vi "LVJSON Flatten.vi"(8 "error in (no error)":errorcluster, 9 "Enums as string? (F)":bool, 10 "Root Path ([]=Root)":string[](array[string]), 11 "Variant in":variant) -> (0 "error out":errorcluster, 3 "Root Element out":T1)   [LabVIEW 2018, in "labview_json.lvlib"]
uses:
  labview_json.lvlib
  <vilib>/Utility/Data Type/NI_Data Type.lvlib
  Element Type.ctl
  <vilib>/Utility/error.llb/Error Cluster From Error Code.vi
  <vilib>/ErrorRing/Error Ring.xnode
  Element.ctl
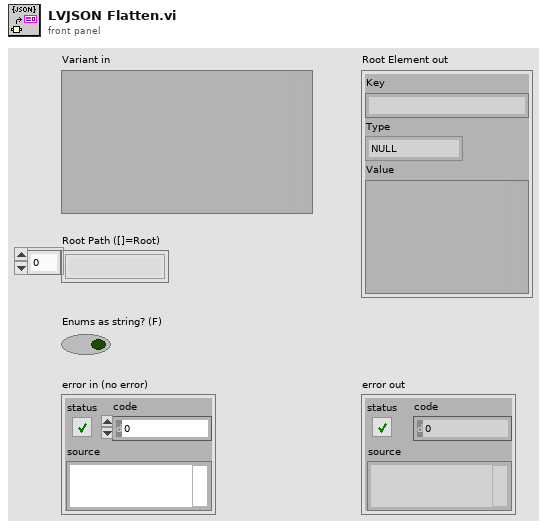
[diagram p1: front panel]
types:
  T1 = typedef "labview_json.lvlib/Element.ctl" = cluster{"Key":string, "Type":T2, "Value":variant}
  T2 = typedef "labview_json.lvlib/Element Type.ctl" = enum8{"NULL", "BOOL", "INT", "UINT", "FLOAT", "STRING", "ARRAY", "OBJECT", "SKIP"}
  T3 = typedef "NI_Data Type.lvlib/Data Type.ctl" = enum8{"Invalid Type", "Void", "I8", "I16", "I32", "I64", "U8", "U16", "U32", "U64", "Single Float", "Double Float", "Extended Float", "Single Complex", "Double Complex", "Extended Complex", "Enum U8", "Enum U16", "Enum U32", "Enum U64", "Single Float With Unit", "Double Float With Unit", "Extended Float With Unit", "Single Complex with Unit", "Double Complex with Unit", "Extended Complex with Unit", "Boolean", "String", "Path", "Picture", "Tag", "Array", "Cluster", "Variant", "LV Variant", "Waveform", "Timestamp", "Digital Waveform", "Digital Data", "ExpressData", "Refnum", "External Data", "VI", "Poly VI", "LabVIEW Class Instance", "Fixed Point", "Set Collection", "Map Collection"}
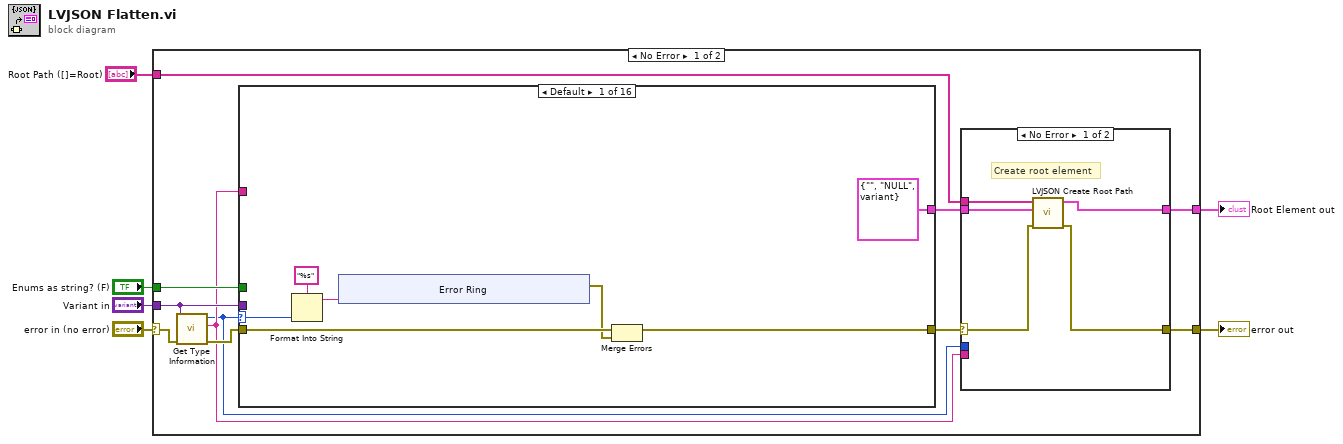
[diagram p0: block diagram]
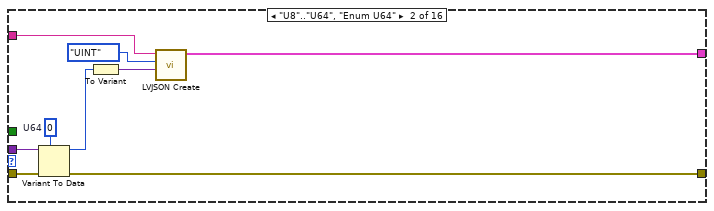
[diagram p2: hidden frame]
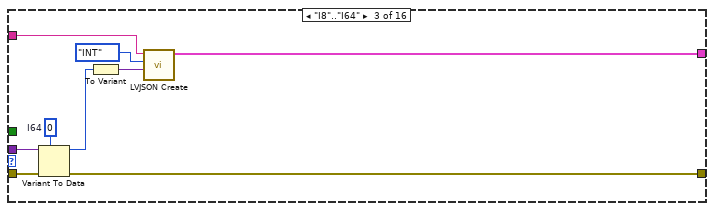
[diagram p3: hidden frame]
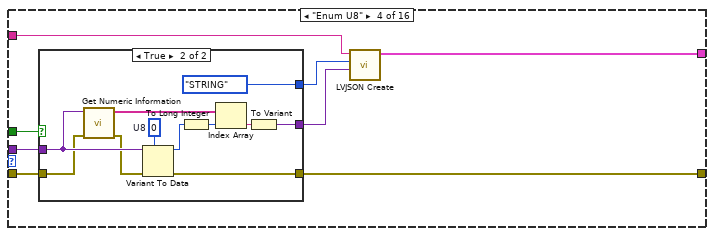
[diagram p4: hidden frame]
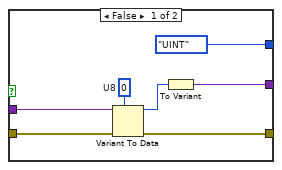
[diagram p5: hidden frame]
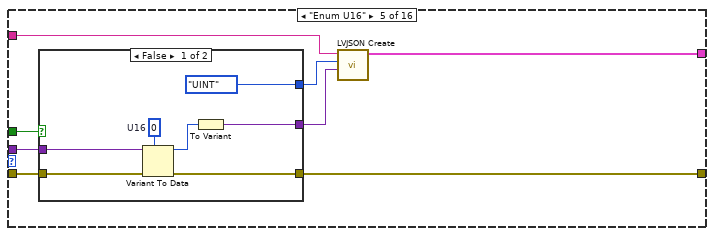
[diagram p6: hidden frame]
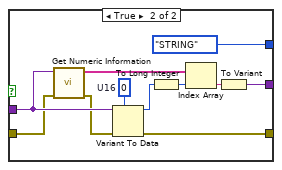
[diagram p7: hidden frame]
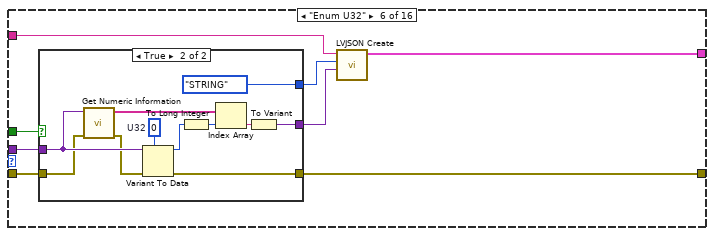
[diagram p8: hidden frame]
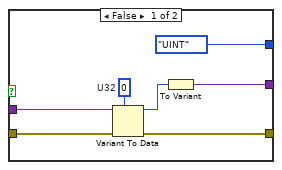
[diagram p9: hidden frame]
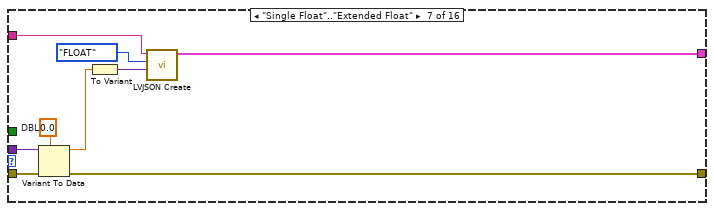
[diagram p10: hidden frame]
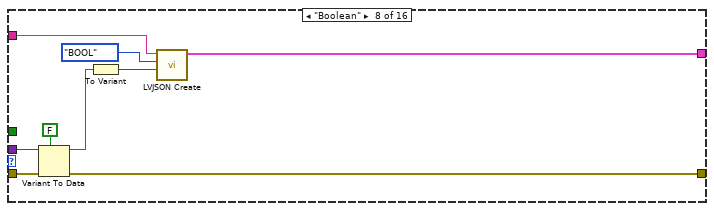
[diagram p11: hidden frame]
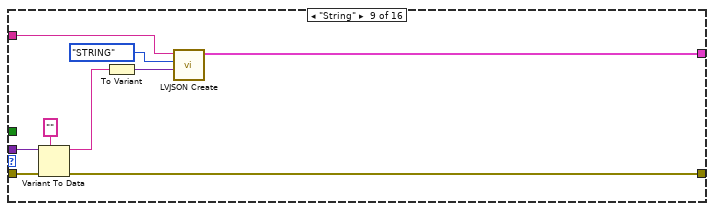
[diagram p12: hidden frame]
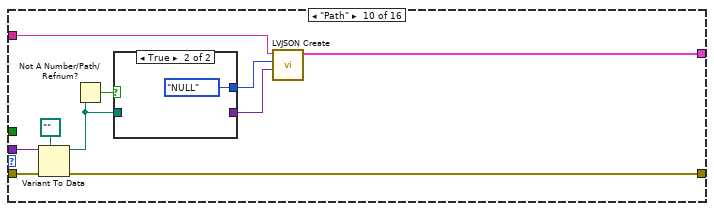
[diagram p13: hidden frame]
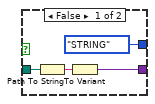
[diagram p14: hidden frame]
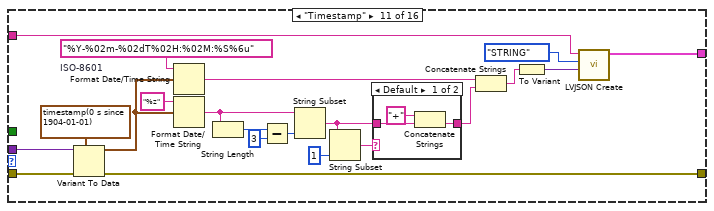
[diagram p15: hidden frame]
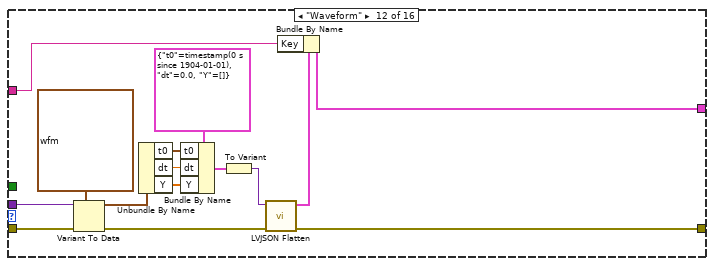
[diagram p17: hidden frame]
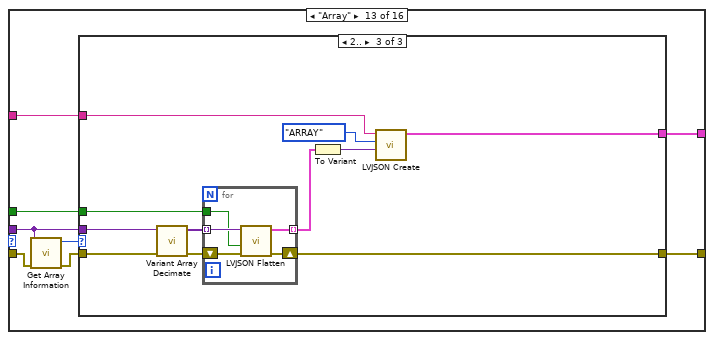
[diagram p18: hidden frame]
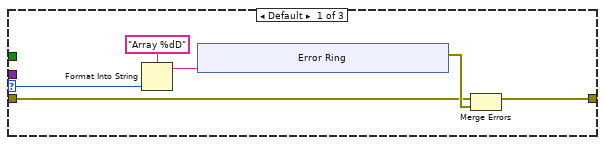
[diagram p19: hidden frame]
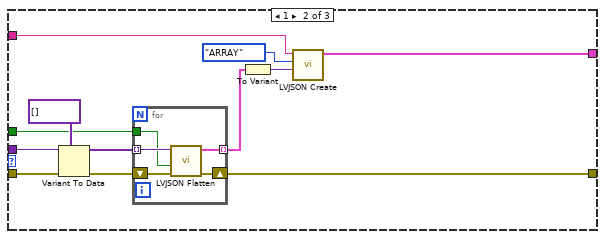
[diagram p20: hidden frame]
diagram:
  n1 = case shown="No Error" "error in (no error)" {
    selector: "error in (no error)" -> [w17 w322]
    tunnel: "Variant in" -> [w15 _]
    tunnel: [w12 w322] -> w4
    tunnel: [w10 _] -> w2
    tunnel: "Enums as string? (F)" -> [w14 _]
    tunnel: "Root Path ([]=Root)" -> [w7 _]
    frame No Error {
      n2 = call <vilib>:"Get Type Information.vi"("error in (no error)"=w17, "variant"=w15) -> ("error out"=w16:errorcluster, "name"=w11:string, "type"=w8:T3)  [unwired: 5 in, 2 out]
      n3 = case shown="Default" w8 {
        selector: w8 -> [w20 _ _ _ _ _ _ _ _ _ _ _ _ _ _ _]
        tunnel: w16 -> [w24 w40 w49 w57 w83 w109 w136 w145 w154 w164 w190 w209 w217 w271 w299 w307]
        tunnel: w15 -> [_ w39 w48 w56 w82 w108 w135 w144 w153 w163 w189 w208 w213 w269 _ w305]
        tunnel: [w23 w37 w46 w55 w81 w107 w133 w143 w152 w162 w188 w200 w214 w273 w299 w301] -> w13
        tunnel: [T1 {"Key"="", "Type"=enum."NULL", "Value"=variant} ("Root Element out") w32 w41 w51 w79 w104 w130 w138 w148 w155 w172 w196 w211 w266 w297 w300] -> w9
        tunnel: w14 -> [_ _ _ w54 w80 w106 _ _ _ _ _ _ w212 w272 _ w302]
        tunnel: w11 -> [_ w35 w42 w50 w76 w105 w131 w140 w149 w158 w173 w195 w210 w267 w298 _]
        frame Default {
          n4 = Format Into String(format string="%s", w20) -> (resulting string=w22:string)  [unwired: 2 in, 1 out]
          n5 = xnode "Error Ring"("parameter 0"=w22) -> ("error out"=w19:errorcluster)
          n6 = Merge Errors(w24, w19) -> (w23:errorcluster)
        }
        frame "U8".."U64", "Enum U64" {
          w38 = u64 0  # U64
          n7 = Variant To Data(error in=w40, type=w38, Variant=w39) -> (data=w36:u64, error out=w37:errorcluster)
          n8 = To Variant(anything=w36) -> (Variant=w33:variant)
          n9 = call "LVJSON Create.vi"("Variant (Void=Default Type)"=w33, "Type"=Element_Type."UINT", "Key"=w35) -> ("Element out"=w32:T1)  [unwired: 8 in]
        }
        frame "I8".."I64" {
          w47 = i64 0  # I64
          n10 = Variant To Data(error in=w49, type=w47, Variant=w48) -> (data=w45:i64, error out=w46:errorcluster)
          n11 = To Variant(anything=w45) -> (Variant=w43:variant)
          n12 = call "LVJSON Create.vi"("Variant (Void=Default Type)"=w43, "Type"=Element_Type."INT", "Key"=w42) -> ("Element out"=w41:T1)  [unwired: 8 in]
        }
        frame "Enum U8" {
          n13 = case shown="True" w54 {
            tunnel: w57 -> [w64 w69]
            tunnel: w56 -> [w63 w73]
            tunnel: [w61 w74] -> w55
            tunnel: [w59 w66] -> w53
            tunnel: [Element_Type."UINT" ("Type") Element_Type."STRING" ("Type")] -> w52
            frame False {
              w62 = u8 0  # U8
              n14 = Variant To Data(error in=w64, type=w62, Variant=w63) -> (data=w60:u8, error out=w61:errorcluster)
              n15 = To Variant(anything=w60) -> (Variant=w59:variant)
            }
            frame True {
              w75 = u8 0  # U8
              n16 = call <vilib>:"Get Numeric Information.vi"("error in (no error)"=w69, "variant"=w73) -> ("error out"=w70:errorcluster, "enum names"=w72:string[])  [unwired: 6 in, 2 out]
              n17 = Variant To Data(error in=w70, type=w75, Variant=w73) -> (data=w71:u8, error out=w74:errorcluster)
              n18 = To Long Integer(number=w71) -> (32bit integer=w68:i32)
              n19 = Index Array(array=w72, index=w68) -> (element=w67:string)
              n20 = To Variant(anything=w67) -> (Variant=w66:variant)
            }
          }
          n21 = call "LVJSON Create.vi"("Variant (Void=Default Type)"=w53, "Type"=w52, "Key"=w50) -> ("Element out"=w51:T1)  [unwired: 8 in]
        }
        frame "Enum U16" {
          n22 = case shown="False" w80 {
            tunnel: w83 -> [w90 w95]
            tunnel: w82 -> [w89 w99]
            tunnel: [w87 w100] -> w81
            tunnel: [w85 w92] -> w78
            tunnel: [Element_Type."UINT" ("Type") Element_Type."STRING" ("Type")] -> w77
            frame False {
              w88 = u16 0  # U16
              n23 = Variant To Data(error in=w90, type=w88, Variant=w89) -> (data=w86:u16, error out=w87:errorcluster)
              n24 = To Variant(anything=w86) -> (Variant=w85:variant)
            }
            frame True {
              w101 = u16 0  # U16
              n25 = call <vilib>:"Get Numeric Information.vi"("error in (no error)"=w95, "variant"=w99) -> ("error out"=w96:errorcluster, "enum names"=w98:string[])  [unwired: 6 in, 2 out]
              n26 = Variant To Data(error in=w96, type=w101, Variant=w99) -> (data=w97:u16, error out=w100:errorcluster)
              n27 = To Long Integer(number=w97) -> (32bit integer=w94:i32)
              n28 = Index Array(array=w98, index=w94) -> (element=w93:string)
              n29 = To Variant(anything=w93) -> (Variant=w92:variant)
            }
          }
          n30 = call "LVJSON Create.vi"("Variant (Void=Default Type)"=w78, "Type"=w77, "Key"=w76) -> ("Element out"=w79:T1)  [unwired: 8 in]
        }
        frame "Enum U32" {
          n31 = case shown="True" w106 {
            tunnel: w109 -> [w116 w121]
            tunnel: w108 -> [w115 w125]
            tunnel: [w113 w126] -> w107
            tunnel: [w111 w118] -> w103
            tunnel: [Element_Type."UINT" ("Type") Element_Type."STRING" ("Type")] -> w102
            frame False {
              w114 = u32 0  # U32
              n32 = Variant To Data(error in=w116, type=w114, Variant=w115) -> (data=w112:u32, error out=w113:errorcluster)
              n33 = To Variant(anything=w112) -> (Variant=w111:variant)
            }
            frame True {
              w127 = u32 0  # U32
              n34 = call <vilib>:"Get Numeric Information.vi"("error in (no error)"=w121, "variant"=w125) -> ("error out"=w122:errorcluster, "enum names"=w124:string[])  [unwired: 6 in, 2 out]
              n35 = Variant To Data(error in=w122, type=w127, Variant=w125) -> (data=w123:u32, error out=w126:errorcluster)
              n36 = To Long Integer(number=w123) -> (32bit integer=w120:i32)
              n37 = Index Array(array=w124, index=w120) -> (element=w119:string)
              n38 = To Variant(anything=w119) -> (Variant=w118:variant)
            }
          }
          n39 = call "LVJSON Create.vi"("Variant (Void=Default Type)"=w103, "Type"=w102, "Key"=w105) -> ("Element out"=w104:T1)  [unwired: 8 in]
        }
        frame "Single Float".."Extended Float" {
          w134 = 0.0  # DBL
          n40 = Variant To Data(error in=w136, type=w134, Variant=w135) -> (data=w132:dbl, error out=w133:errorcluster)
          n41 = To Variant(anything=w132) -> (Variant=w129:variant)
          n42 = call "LVJSON Create.vi"("Variant (Void=Default Type)"=w129, "Type"=Element_Type."FLOAT", "Key"=w131) -> ("Element out"=w130:T1)  [unwired: 8 in]
        }
        frame "Boolean" {
          n43 = Variant To Data(error in=w145, type=FALSE, Variant=w144) -> (data=w141:bool, error out=w143:errorcluster)
          n44 = To Variant(anything=w141) -> (Variant=w137:variant)
          n45 = call "LVJSON Create.vi"("Variant (Void=Default Type)"=w137, "Type"=Element_Type."BOOL", "Key"=w140) -> ("Element out"=w138:T1)  [unwired: 8 in]
        }
        frame "String" {
          n46 = Variant To Data(error in=w154, type="", Variant=w153) -> (data=w150:string, error out=w152:errorcluster)
          n47 = To Variant(anything=w150) -> (Variant=w147:variant)
          n48 = call "LVJSON Create.vi"("Variant (Void=Default Type)"=w147, "Type"=Element_Type."STRING", "Key"=w149) -> ("Element out"=w148:T1)  [unwired: 8 in]
        }
        frame "Path" {
          n49 = Variant To Data(error in=w164, type=path "", Variant=w163) -> (data=w160:path, error out=w162:errorcluster)
          n50 = Not A Number/Path/Refnum?(number/path/refnum=w160) -> (NaN/Path/Refnum?=w159:bool)
          n51 = case shown="True" w159 {
            tunnel: [w166 _] -> w156
            tunnel: w160 -> [w168 _]
            tunnel: [Element_Type."STRING" ("Type") Element_Type."NULL" ("Type")] -> w157
            frame False {
              n52 = Path To String(path=w168) -> (string=w167:string)
              n53 = To Variant(anything=w167) -> (Variant=w166:variant)
            }
            frame True {
            }
          }
          n54 = call "LVJSON Create.vi"("Variant (Void=Default Type)"=w156, "Type"=w157, "Key"=w158) -> ("Element out"=w155:T1)  [unwired: 8 in]
        }
        frame "Timestamp" {
          w186 = "%Y-%02m-%02dT%02H:%02M:%S%6u"  # ISO-8601
          n55 = Variant To Data(error in=w190, type=timestamp(0 s since 1904-01-01), Variant=w189) -> (data=w175:timestamp, error out=w188:errorcluster)
          n56 = Format Date/Time String(time format string (%c)=w186, seconds (now)=w175) -> (date/time string=w185:string)  [unwired: 1 in]
          n57 = Format Date/Time String(time format string (%c)="%z", seconds (now)=w175) -> (date/time string=w183:string)  [unwired: 1 in]
          n58 = String Length(string=w183) -> (length=w182:i32)
          n59 = Subtract(x=w182, y=3) -> (x-y=w180:i32)
          n60 = String Subset(string=w183, length (rest)=w180) -> (substring=w177:string)  [unwired: 1 in]
          n61 = String Subset(string=w177, length (rest)=1 ("length (rest)")) -> (substring=w178:string)  [unwired: 1 in]
          n62 = case shown="Default" w178 {
            tunnel: [w192 w194] -> w176
            tunnel: w177 -> [w193 w194]
            frame Default {
              n63 = Concatenate Strings("+" ("string"), w193) -> (w192:string)
            }
            frame "-" {
            }
          }
          n64 = Concatenate Strings(w185, w176) -> (w174:string)
          n65 = To Variant(anything=w174) -> (Variant=w171:variant)
          n66 = call "LVJSON Create.vi"("Variant (Void=Default Type)"=w171, "Type"=Element_Type."STRING", "Key"=w173) -> ("Element out"=w172:T1)  [unwired: 8 in]
        }
        frame "Waveform" {
          n67 = Variant To Data(error in=w209, type=waveform(dbl) {"t0"=timestamp(0 s since 1904-01-01), "dt"=1.0, "Y"=[]} ("Waveform"), Variant=w208) -> (data=w205:waveform(dbl), error out=w201:errorcluster)
          n68 = Unbundle By Name(w205) -> ("t0"=w204:timestamp, "dt"=w203:dbl, "Y"=w202:dbl[])
          n69 = Bundle By Name(cluster=cluster{"t0":timestamp, "dt":dbl, "Y":dbl[]} {"t0"=timestamp(0 s since 1904-01-01), "dt"=0.0, "Y"=[]} ("Waveform"), "t0"=w204, "dt"=w203, "Y"=w202) -> (w199:cluster{"t0":timestamp, "dt":dbl, "Y":dbl[]})
          n70 = To Variant(anything=w199) -> (Variant=w198:variant)
          n71 = call "LVJSON Flatten.vi"("error in (no error)"=w201, "Variant in"=w198) -> ("error out"=w200:errorcluster, "Root Element out"=w197:T1)  [unwired: 8 in]
          n72 = Bundle By Name(cluster=w197, "Key"=w195) -> (w196:T1)
        }
        frame "Array" {
          n73 = call <vilib>:"Get Array Information.vi"("error in (no error)"=w217, "variant"=w213) -> ("error out"=w215:errorcluster, "number of dimensions"=w216:i32)  [unwired: 6 in, 2 out]
          n74 = case shown="2.." w216 {
            selector: w216 -> [w218 _ _]
            tunnel: w215 -> [w220 w242 w254]
            tunnel: [w219 w236 w257] -> w214
            tunnel: w213 -> [_ w241 w255]
            tunnel: w212 -> [_ w237 w258]
            tunnel: [_ w231 w248] -> w211
            tunnel: w210 -> [_ w234 w249]
            frame Default {
              n75 = Format Into String(format string="Array %dD", w218) -> (resulting string=w223:string)  [unwired: 2 in, 1 out]
              n76 = xnode "Error Ring"("parameter 0"=w223) -> ("error out"=w221:errorcluster)
              n77 = Merge Errors(w220, w221) -> (w219:errorcluster)
            }
            frame 1 {
              n78 = Variant To Data(error in=w242, type=variant[] [], Variant=w241) -> (data=w238:variant[], error out=w239:errorcluster)
              n79 = for {
                tunnel: w238 -> [w246] mode=indexing
                tunnel: w237 -> [w243]
                shift-right: [w245] -> w236
                shift-left: w239 -> [w247]
                tunnel: [w244] -> w235 mode=indexing
                n80 = call "LVJSON Flatten.vi"("error in (no error)"=w247, "Enums as string? (F)"=w243, "Variant in"=w246) -> ("error out"=w245:errorcluster, "Root Element out"=w244:T1)  [unwired: 7 in]
              }
              n81 = To Variant(anything=w235) -> (Variant=w232:variant)
              n82 = call "LVJSON Create.vi"("Variant (Void=Default Type)"=w232, "Type"=Element_Type."ARRAY", "Key"=w234) -> ("Element out"=w231:T1)  [unwired: 8 in]
            }
            frame 2.. {
              n83 = call "Variant Array Decimate.vi"("error in (no error)"=w254, "N Dim Array"=w255) -> ("error out"=w253:errorcluster, "Array of Variant Arrays"=w252:variant[])  [unwired: 6 in, 2 out]
              n84 = for {
                tunnel: w252 -> [w262] mode=indexing
                tunnel: w258 -> [w259]
                shift-right: [w261] -> w257
                shift-left: w253 -> [w263]
                tunnel: [w260] -> w256 mode=indexing
                n85 = call "LVJSON Flatten.vi"("error in (no error)"=w263, "Enums as string? (F)"=w259, "Variant in"=w262) -> ("error out"=w261:errorcluster, "Root Element out"=w260:T1)  [unwired: 7 in]
              }
              n86 = To Variant(anything=w256) -> (Variant=w251:variant)
              n87 = call "LVJSON Create.vi"("Variant (Void=Default Type)"=w251, "Type"=Element_Type."ARRAY", "Key"=w249) -> ("Element out"=w248:T1)  [unwired: 8 in]
            }
          }
        }
        frame "Cluster" {
          n88 = call "Variant Is LVJSON.vi"("Variant"=w269) -> ("Is LVJSON?"=w268:bool)
          n89 = case shown="False" w268 {
            tunnel: [w279 w294] -> w273
            tunnel: w272 -> [w278 _]
            tunnel: w271 -> [w277 w294]
            tunnel: [w276 _] -> w270
            tunnel: w269 -> [w275 _]
            frame False {
              n90 = call "Variant Is Empty Object.vi"("Variant"=w275) -> ("Is Empty Object?"=w274:bool)
              n91 = case shown="False" w274 {
                tunnel: [w287 w293] -> w279
                tunnel: w278 -> [w286 _]
                tunnel: w277 -> [w283 w293]
                tunnel: [w282 _] -> w276
                tunnel: w275 -> [w281 _]
                frame False {
                  n92 = Variant To Data(error in=w283, type=variant[] [], Variant=w281) -> (data=w280:variant[], error out=w284:errorcluster)
                  n93 = for {
                    tunnel: w280 -> [w291] mode=indexing
                    tunnel: w286 -> [w288]
                    shift-right: [w290] -> w287
                    shift-left: w284 -> [w292]
                    tunnel: [w289] -> w282 mode=indexing
                    n94 = call "LVJSON Flatten.vi"("error in (no error)"=w292, "Enums as string? (F)"=w288, "Variant in"=w291) -> ("error out"=w290:errorcluster, "Root Element out"=w289:T1)  [unwired: 7 in]
                  }
                }
                frame True {
                  # "Empty object"
                }
              }
            }
            frame True {
              # "Is LVJSON Cluster"
            }
          }
          n95 = To Variant(anything=w270) -> (Variant=w265:variant)
          n96 = call "LVJSON Create.vi"("Variant (Void=Default Type)"=w265, "Type"=Element_Type."OBJECT", "Key"=w267) -> ("Element out"=w266:T1)  [unwired: 8 in]
        }
        frame "Void" {
          # "Void or LV Variant are NULL\nsince empty arrays return Void types"
          n97 = call "LVJSON Create.vi"("Variant (Void=Default Type)"=variant ("Value"), "Type"=Element_Type."NULL", "Key"=w298) -> ("Element out"=w297:T1)  [unwired: 8 in]
        }
        frame "LV Variant" {
          n98 = Variant To Data(error in=w307, type=variant, Variant=w305) -> (data=w303:variant, error out=w306:errorcluster)
          n99 = call "LVJSON Flatten.vi"("error in (no error)"=w306, "Enums as string? (F)"=w302, "Variant in"=w303) -> ("error out"=w301:errorcluster, "Root Element out"=w300:T1)  [unwired: 7 in]
        }
      }
      n100 = case shown="No Error" w13 {
        selector: w13 -> [w311 w316]
        tunnel: [w310 w315] -> w12
        tunnel: w8 -> [_ w314]
        tunnel: w11 -> [_ w313]
        tunnel: [w309 _] -> w10
        tunnel: w9 -> [w308 _]
        tunnel: w7 -> [w312 _]
        frame No Error {
          # "Create root element"
          n101 = call "LVJSON Create Root Path.vi"("error in (no error)"=w311, "Element in"=w308, "Root Path"=w312) -> ("error out"=w310:errorcluster, "Root Element out"=w309:T1)  [unwired: 7 in]
        }
        frame Error {
          n102 = in-place {
            in-place-border: w314 -> [w318]
            in-place-border: w313 -> [w317]
            n103 = in-place-cluster #1(w316) -> ("source"=w321:string)
            n104 = Format Into String(format string="\n\nType: %s\nName: %s", initial string=w321, w318, w317) -> (resulting string=w320:string)  [unwired: 1 in, 1 out]
            n105 = in-place-cluster #1("source"=w320) -> (w315:errorcluster)
          }
        }
      }
    }
    frame Error {
    }
  }
  "error out" <- w4
  "Root Element out" <- w2
